vi "Target - HTTP Get for Async Call.vi"(10 "Remote Port":u16=80, 11 "Address":string) -> (3 "Results":string)   [LabVIEW 2023]
doc: "Send an HTTP Get request to the specified address."
panel:
  out "error out":errorcluster
  # "This VI is used by the Benchmarking Asynchronous Calls.vi."
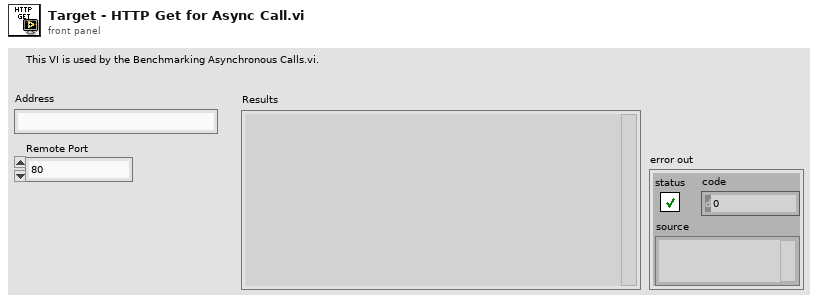
[diagram p1: front panel]
types:
  T1 = enum16{"Standard", "Buffered", "CRLF", "Immediate"}
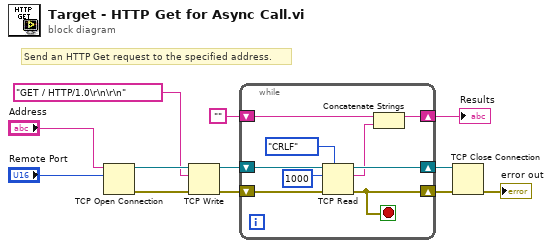
[diagram p0: block diagram]
diagram:
  # "Send an HTTP Get request to the specified address."
  n1 = TCP Open Connection(address="Address", remote port or service name="Remote Port") -> (connection ID=w9:refnum<k5>, error out=w10:errorcluster)  [unwired: 3 in]
  n2 = TCP Write(connection ID=w9, data in="GET / HTTP/1.0\r\n\r\n" ("URI"), error in (no error)=w10) -> (connection ID out=w8:refnum<k5>, error out=w7:errorcluster)  [unwired: 1 in, 1 out]
  n3 = while {
    shift-right: [w19] -> w3
    shift-left: w8 -> [w21]
    shift-right: [w13] -> w4
    shift-left: w7 -> [w20]
    shift-right: [w15] -> w5
    shift-left: "" -> [w14]
    stop <- w13 stop-if-true
    n4 = TCP Read(connection ID=w21, bytes to read=1000, error in (no error)=w20, 7:T1."CRLF" ("mode (standard)")) -> (connection ID out=w19:refnum<k5>, data out=w16:string, error out=w13:errorcluster)  [unwired: 1 in]
    n5 = Concatenate Strings(w14, w16) -> (w15:string)
  }
  "Results" <- w5
  n6 = TCP Close Connection(connection ID=w3, error in (no error)=w4) -> (error out=→"error out":errorcluster)  [unwired: 1 in, 1 out]
